vi "FindStats.vi"(7 "Actor":refnum<class "Actor.lvclass">) -> (3 "Stats":T1)   [LabVIEW 2020, in "jettl.lvlib" / "Base.lvlib" / "Actor.lvclass"]
uses:
  Actor.lvclass
  Actor.lvclass/Actor.ctl
  C:/Users/nathan.davis/Desktop/personal/jettl-harness/repos/jettl/src/jettl/jettl/Base/Actor/Actor.lvclass
  C:/Users/nathan.davis/Desktop/personal/jettl-harness/repos/jettl/src/jettl/jettl/Actor/Actor.lvclass
  jettl.lvlib
  Msg/Msg.lvclass
  MsgSet.ctl
  Stats.ctl
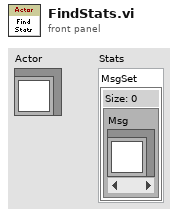
[diagram p1: front panel]
types:
  T1 = typedef "jettl.lvlib/Stats.ctl" = cluster{"MsgSet":T2}
  T2 = typedef "jettl.lvlib/MsgSet.ctl" = set{refnum<class "Msg.lvclass">}
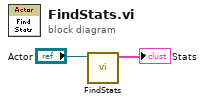
[diagram p0: block diagram]
diagram:
  n1 = call "FindStats.vi"("Actor.lvclass"="Actor") -> ("Stats"=→"Stats":T1)  [unwired: 10 in]
